vi "SinC Wave Chart [While loop].vi"() -> ()   [LabVIEW 2017]
panel:
  in  "stop":bool
  out "Sinc Plot":dbl(graph)
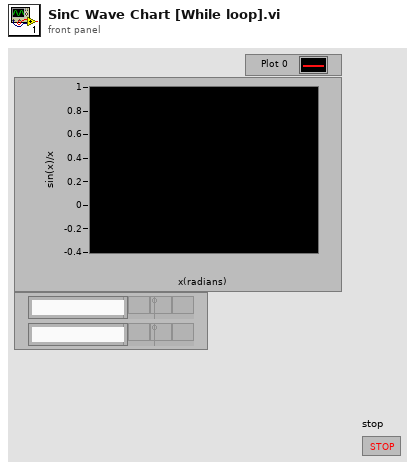
[diagram p1: front panel]
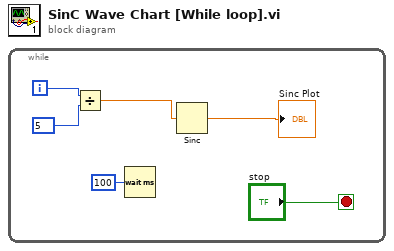
[diagram p0: block diagram]
diagram:
  n1 = while {
    i -> [w4]
    stop <- "stop" stop-if-true
    n2 = Divide(x=w4, y=5) -> (x/y=w2:dbl)
    n3 = Wait (ms)(milliseconds to wait=u32 100) -> ()  [unwired: 1 out]
    n4 = Sinc(1:w2) -> (0:→"Sinc Plot":dbl)
  }
